vi "StringToNumber.vi"(11 "read buffer":string) -> (3 "Numeric":i32)   [LabVIEW 2022 SP3]
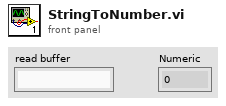
[diagram p1: front panel]
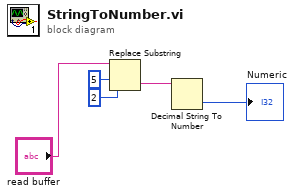
[diagram p0: block diagram]
diagram:
  n1 = Replace Substring(2:2 ("length (len. of substring)"), 3:5 ("offset (0)"), 5:"read buffer") -> (0:w4:string)  [unwired: 1 in, 1 out]
  n2 = Decimal String To Number(string=w4) -> (number=→"Numeric":i32)  [unwired: 2 in, 1 out]
